vi "Set Y Max.vi"(7 "# Elem":dbl, 10 "Array":dbl[](array[numeric]), 11 "XYGraph in":refnum<vi>) -> (3 "# Elem Out":dbl)   [LabVIEW 2012]
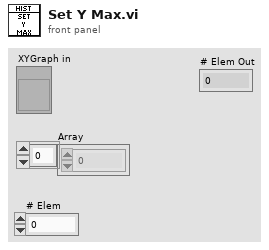
[diagram p1: front panel]
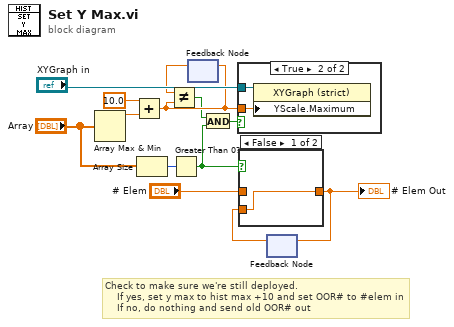
[diagram p0: block diagram]
diagram:
  # "Check to make sure we're still deployed.\n    If yes, set y max to hist max +10 and set OOR# to #elem in\n    If no, do nothing and send old OOR# out"
  n1 = Array Max & Min(array="Array") -> (max value=w9:dbl)  [unwired: 3 out]
  n2 = Add(x=10.0, y=w9) -> (x+y=w11:dbl)
  n3 = Array Size(array="Array") -> (size(s)=w5:i32)
  n4 = Greater Than 0?(x=w5) -> (x > 0?=w4:bool)
  n5 = feedback #1() -> (w12:dbl)  [unwired: 1 in]
  n6 = Not Equal?(x=w12, y=w11) -> (x != y?=w7:bool)
  n7 = feedback-in #1(w11) -> ()
  n8 = And(x=w7, y=w4) -> (x .and. y?=w8:bool)
  n9 = case shown="True" w8 {
    tunnel: w11 -> [_ w15]
    tunnel: "XYGraph in" -> [_ w14]
    frame False {
    }
    frame True {
      n10 = property on="Property Node" class="XYGraph (strict)"(reference=w14, "YScale.Maximum"=w15) -> ()  [unwired: 1 in, 2 out]
    }
  }
  n11 = feedback #2() -> (w2:dbl)  [unwired: 1 in]
  n12 = case shown="False" w4 {
    tunnel: "# Elem" -> [_ w17]
    tunnel: [w16 w17] -> w1
    tunnel: w2 -> [w16 _]
    frame False {
    }
    frame True {
    }
  }
  "# Elem Out" <- w1
  n13 = feedback-in #2(w1) -> ()
